vi "StopControl.vi"(6 "SubPanels":refnum<vi>[](array[refnum]), 8 "WindowButton":refnum<vi>, 9 "StopButton":refnum<vi>, 11 "Plugin Info":T1) -> ()   [LabVIEW 2016]
uses:
  CorePluginInfo.ctl
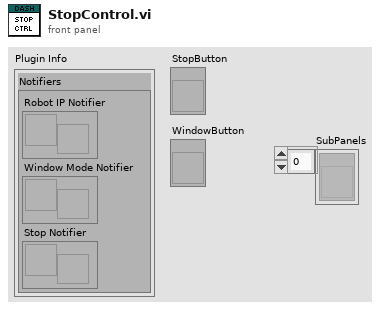
[diagram p1: front panel]
types:
  T1 = typedef "CorePluginInfo.ctl" = cluster{"Notifiers":cluster{"Robot IP Notifier":refnum<notifier>, "Window Mode Notifier":refnum<notifier>, "Stop Notifier":refnum<notifier>}}
  T2 = enum32{"Bad", "Idle", "Run top level", "Running"}
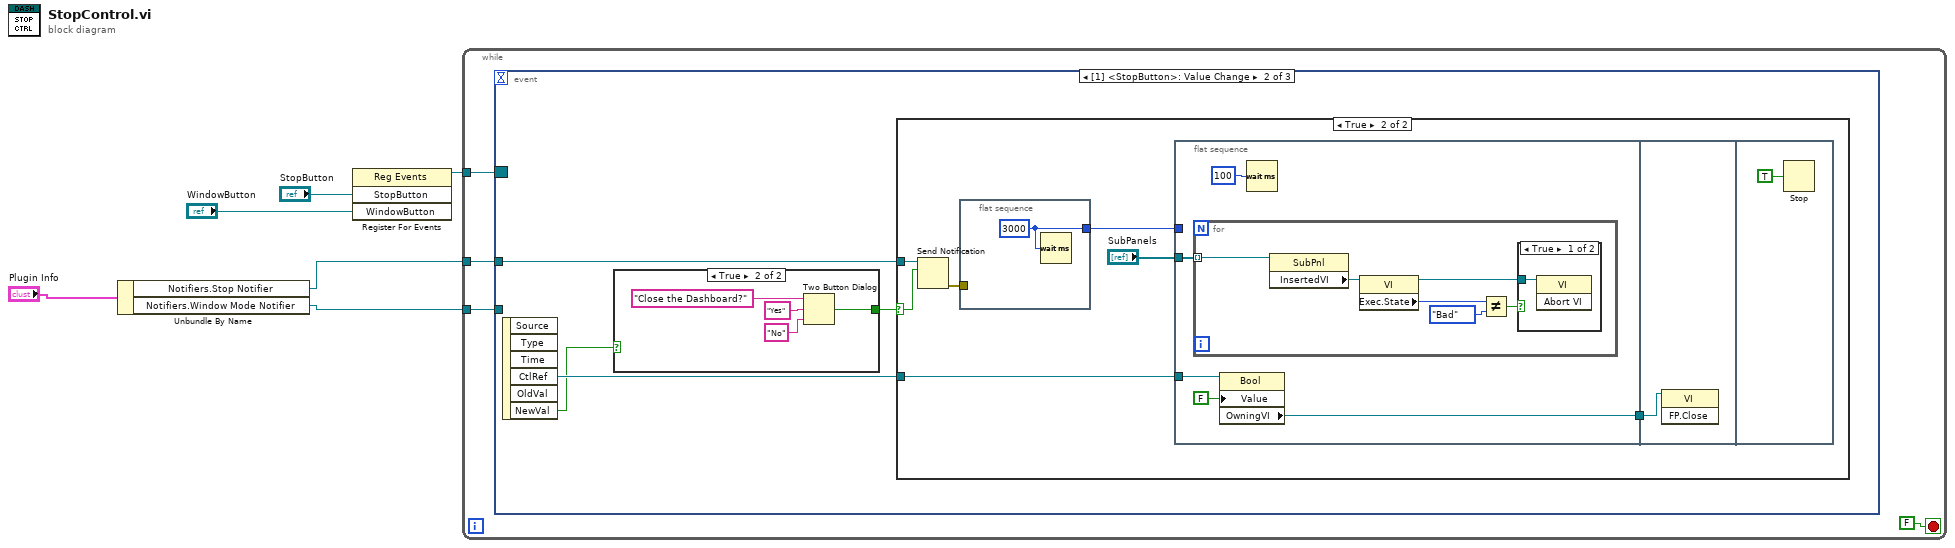
[diagram p0: block diagram]
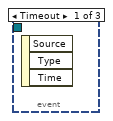
[diagram p2: hidden frame]
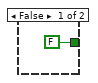
[diagram p3: hidden frame]
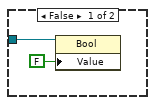
[diagram p4: hidden frame]
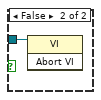
[diagram p5: hidden frame]
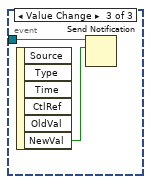
[diagram p6: hidden frame]
diagram:
  n1 = Unbundle By Name("Plugin Info") -> ("Notifiers.Stop Notifier"=w1:refnum<notifier>, "Notifiers.Window Mode Notifier"=w2:refnum<notifier>)
  n2 = register-events("StopButton", "WindowButton") -> (reference out=w5:refnum<event-registration>)  [unwired: 2 in, 1 out]
  n3 = while {
    tunnel: w2 -> [w9]
    tunnel: w1 -> [w8]
    tunnel: w5 -> [w7]
    stop <- FALSE stop-if-true
    n4 = event shown="[1] <StopButton>: Value Change" {
      selector: w7 -> [_ _ _]
      dyn-events: _ -> [_ _ _]
      timeout: _ -> [_ _ _]
      tunnel: w9 -> [_ _ w46]
      tunnel: w8 -> [_ w14 _]
      event Timeout {
        n5 = event-data() -> ()  [unwired: 1 in, 3 out]
      }
      event Value Change {
        n6 = event-data() -> ("CtlRef"=w13:refnum<vi>, "NewVal"=w12:bool)  [unwired: 1 in, 4 out]
        n7 = case shown="True" w12 {
          tunnel: [FALSE ("T button?") w16] -> w11
          frame False {
          }
          frame True {
            n8 = Two Button Dialog(message="Close the Dashboard?", 1:"No" ("F button name (\"Cancel\")"), 2:"Yes" ("T button name (\"OK\")")) -> (T button?=w16:bool)
          }
        }
        n9 = case shown="True" w11 {
          selector: w11 -> [_ w23]
          tunnel: w14 -> [_ w27]
          tunnel: w13 -> [w21 w24]
          frame False {
            n10 = property class="Bool"(reference=w21, "Value"=FALSE) -> ()  [unwired: 1 in, 2 out]
          }
          frame True {
            n11 = Send Notification(notification=w23, notifier=w27) -> (error out=w26:errorcluster)  [unwired: 1 in, 1 out]
            n12 = flat-sequence {
              tunnel: w26 -> [_]
              tunnel: [w29] -> w25
              frame #0 {
                w29 = u32 3000 ("milliseconds to wait")
                n13 = Wait (ms)(milliseconds to wait=w29) -> ()  [unwired: 1 out]
              }
            }
            n14 = flat-sequence {
              tunnel: w25 -> [_]
              tunnel: w24 -> [w33]
              tunnel: [w31] -> w28
              tunnel: "SubPanels" -> [w30]
              tunnel: w28 -> [w43]
              frame #0 {
                n15 = for {
                  tunnel: w30 -> [w40] mode=indexing
                  n16 = property class="SubPnl"(reference=w40) -> ("InsertedVI"=w39:refnum<vi>)  [unwired: 1 in, 2 out]
                  n17 = property class="VI"(reference=w39) -> (reference out=w35:refnum<vi>, "Exec.State"=w38:T2)  [unwired: 1 in, 1 out]
                  n18 = Not Equal?(x=w38, y=T2."Bad") -> (x != y?=w36:bool)
                  n19 = case shown="True" w36 {
                    tunnel: w35 -> [w41 w42]
                    frame True {
                      n20 = invoke class="VI" method="Abort VI"(reference=w41) -> ()  [unwired: 2 in, 3 out]
                    }
                    frame False {
                      n21 = invoke class="VI" method="Abort VI"(reference=w42) -> ()  [unwired: 2 in, 3 out]
                    }
                  }
                }
                n22 = property class="Bool"(reference=w33, "Value"=FALSE) -> ("OwningVI"=w31:refnum<vi>)  [unwired: 1 in, 2 out]
                n23 = Wait (ms)(milliseconds to wait=u32 100) -> ()  [unwired: 1 out]
              }
              frame #1 {
                n24 = invoke class="VI" method="FP.Close"(reference=w43) -> ()  [unwired: 2 in, 3 out]
              }
              frame #2 {
                n25 = Stop(stop? (T)=TRUE) -> ()
              }
            }
          }
        }
      }
      event Value Change {
        n26 = event-data() -> ("NewVal"=w45:bool)  [unwired: 1 in, 5 out]
        n27 = Send Notification(notification=w45, notifier=w46) -> ()  [unwired: 1 in, 2 out]
      }
    }
  }
